vi "Call HTML Help Generation Functions Async.vi"(8 "error in (no error)":errorcluster, 9 "Extra Page Names":string[](array[string]), 11 "Destination Base Path":path) -> (0 "error out":errorcluster, 3 "Destination Base Path Out (dup)":path)   [LabVIEW 2015, in "NIVS_Consolidated_CDW_MetaDataObj.lvclass"]
doc: "Call the Copy and Create HTML file functions."
uses:
  NIVS_Consolidated_CDW_MetaDataObj.lvclass
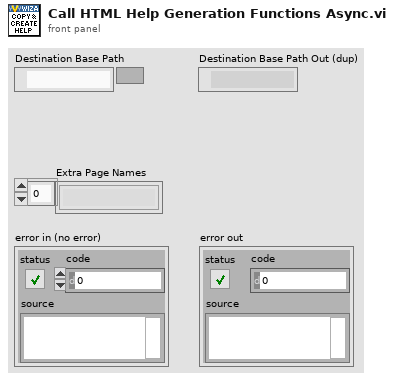
[diagram p1: front panel]
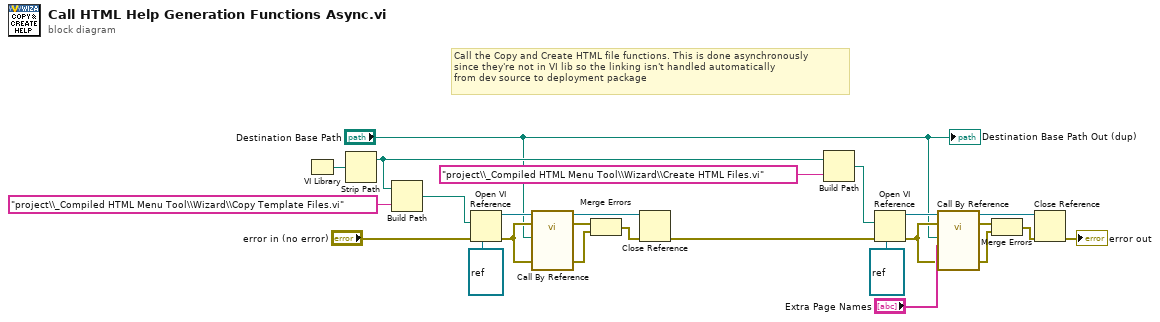
[diagram p0: block diagram]
diagram:
  # "Call the Copy and Create HTML file functions. This is done asynchronously\nsince they're not in VI lib so the linking isn't handled automatically\nfrom dev source to deployment package"
  n1 = VI Library() -> (path=w2:path)
  n2 = Strip Path(path=w2) -> (stripped path=w12:path)  [unwired: 1 out]
  n3 = Build Path(base path=w12, name or relative path="project\\_Compiled HTML Menu Tool\\Wizard\\Copy Template Files.vi") -> (appended path=w4:path)
  n4 = Open VI Reference(type specifier VI Refnum (for type only)=refnum<vi> refnum, vi path=w4, error in (no error)="error in (no error)") -> (vi reference=w6:refnum<vi>, error out=w7:errorcluster)  [unwired: 3 in]
  n5 = call-by-ref "?"(reference=w6, error in=w7, 8:"error in (no error)"=w7, "Base Path"="Destination Base Path") -> (reference out=w11:refnum<vi>, error out=w8:errorcluster, 0:"error out"=w9:errorcluster)  [unwired: 9 in]
  n6 = Merge Errors(w8, w9) -> (w10:errorcluster)
  n7 = Close Reference(reference=w11, error in (no error)=w10) -> (error out=w25:errorcluster)
  n8 = Build Path(base path=w12, name or relative path="project\\_Compiled HTML Menu Tool\\Wizard\\Create HTML Files.vi") -> (appended path=w15:path)
  n9 = Open VI Reference(type specifier VI Refnum (for type only)=refnum<vi> refnum, vi path=w15, error in (no error)=w25) -> (vi reference=w17:refnum<vi>, error out=w18:errorcluster)  [unwired: 3 in]
  n10 = call-by-ref "?"(reference=w17, error in=w18, 8:"error in (no error)"=w18, "Topics"="Extra Page Names", "path"="Destination Base Path") -> (reference out=w21:refnum<vi>, error out=w22:errorcluster, 0:"error out"=w23:errorcluster)  [unwired: 8 in]
  n11 = Merge Errors(w22, w23) -> (w20:errorcluster)
  n12 = Close Reference(reference=w21, error in (no error)=w20) -> (error out=→"error out":errorcluster)
  "Destination Base Path Out (dup)" <- "Destination Base Path"
